vi "Get Validate.vi"(11 "PCAN-USB Base Strategy in":refnum<class "PCAN Base Strategy.lvclass">) -> (2 "Validate?":bool, 3 "PCAN-USB Base Strategy out":refnum<class "PCAN Base Strategy.lvclass">)   [LabVIEW 2025, in "PCAN Base Strategy.lvclass"]
uses:
  PCAN Base Strategy.lvclass
  PCAN Base Strategy.lvclass/PCAN Base Strategy.ctl
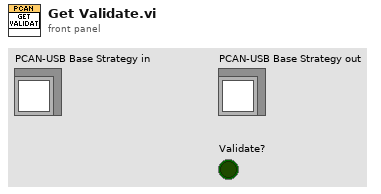
[diagram p1: front panel]
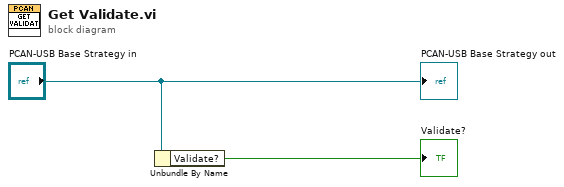
[diagram p0: block diagram]
diagram:
  n1 = Unbundle By Name("PCAN-USB Base Strategy in") -> ("Validate?"=→"Validate?":bool)
  "PCAN-USB Base Strategy out" <- "PCAN-USB Base Strategy in"
